vi "Read Step Data (Manual Mode).vi"(0 "VISA resource name":refnum<visa-resource-name>, 5 "Step (1)":i32=1 min=1 max=9 step=1 format="%2_0f", 11 "error in (no error)":errorcluster) -> (4 "VISA resource name out":refnum<visa-resource-name>, 6 "Test Meter Data Output":T1 {"Frequency (Hz)" format="%.1f"; "Voltage (V)" format="%.1f"; "RMS Current (A)" format="%.3f"; "Power (W)" format="%.1f"; "Peak Current (A)" format="%.1f"; "Power Factor" format="%.3f"}, 15 "error out":errorcluster)   [LabVIEW 2020]
doc: "Reads the Manual mode <B>Step data</B>. \n\nIn Manual Mode the output data cluster has the following data.\n\n1. Memory\n2. Frequency (Hz)\n3. Voltage (V)\n4. RMS Current (A)\n5. Peak Current (A)\n6. Power (W)\n7. Power Factor\n8. Status\n\nNote: This setting is supported for <B>Firmware Version 2.0</B> Only"
uses:
  <instrlib>/eec 6700/eec 6700.lvlib
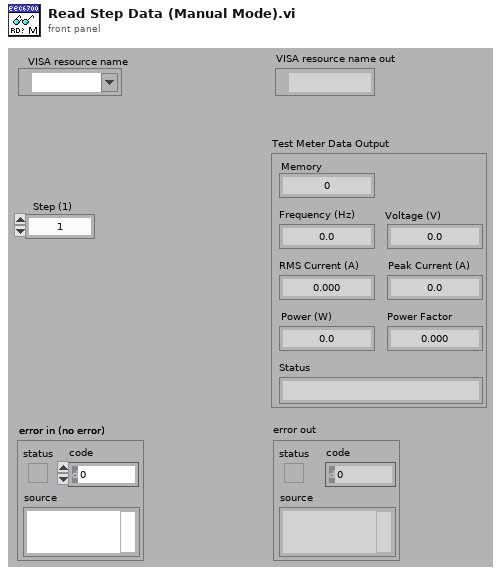
[diagram p1: front panel]
types:
  T1 = cluster{"Memory":i32, "Frequency (Hz)":dbl, "Voltage (V)":dbl, "RMS Current (A)":dbl, "Peak Current (A)":dbl, "Power (W)":dbl, "Power Factor":dbl, "Status":string}
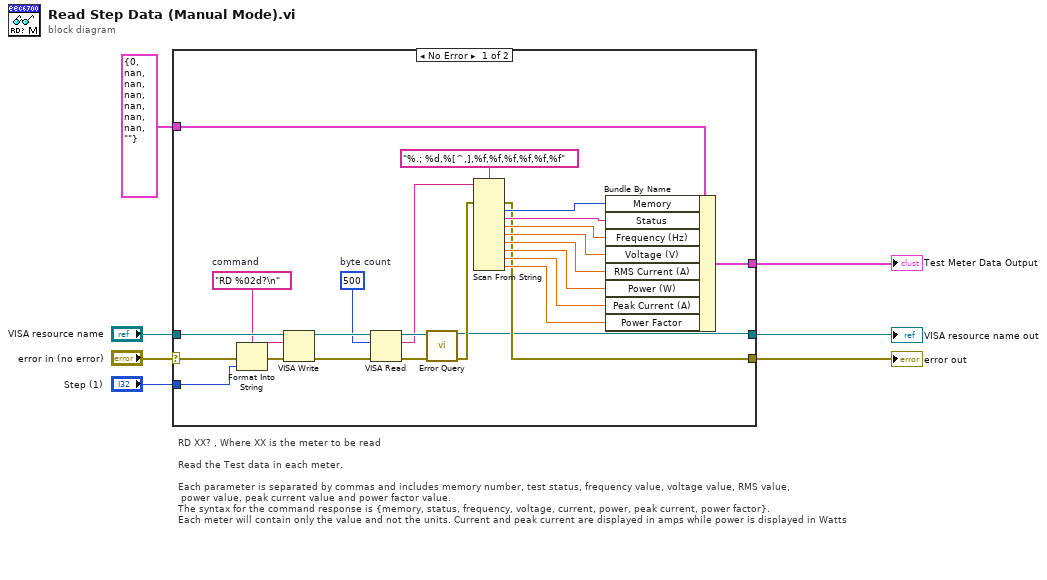
[diagram p0: block diagram]
diagram:
  # "RD XX? , Where XX is the meter to be read\n\nRead the Test data in each meter. \n\nEach parameter is separated by commas and includes memory number, test status, frequency value, voltage value, RMS value,\n power value, peak current value and power factor value. \nThe syntax for the command response is {memory, status, frequency, voltage, current, power, peak current, power factor}. \nEach meter will contain only the value and not the units. Current and peak current are displayed in amps while power is displayed in Watts"
  n1 = case shown="No Error" "error in (no error)" {
    selector: "error in (no error)" -> [w29 w35]
    tunnel: "VISA resource name" -> [w30 w36]
    tunnel: [w9 w36] -> w5
    tunnel: [w12 w35] -> w4
    tunnel: [w8 w34] -> w2
    tunnel: T1 {"Memory"=0, "Frequency (Hz)"=nan, "Voltage (V)"=nan, "RMS Current (A)"=nan, "Peak Current (A)"=nan, "Power (W)"=nan, "Power Factor"=nan, "Status"=""} ("Test Meter Data Output") -> [w10 w34]
    tunnel: "Step (1)" -> [w23 _]
    frame No Error {
      w25 = "RD %02d?\n"  # command
      w31 = u32 500  # byte count
      n2 = Format Into String(format string=w25, error in=w29, w23) -> (resulting string=w24:string, error out=w26:errorcluster)  [unwired: 1 in]
      n3 = VISA Write(VISA resource name=w30, write buffer=w24, error in (no error)=w26) -> (VISA resource name out=w33:refnum<visa-resource-name>, error out=w32:errorcluster)  [unwired: 1 out]
      n4 = VISA Read(VISA resource name=w33, byte count=w31, error in (no error)=w32) -> (VISA resource name out=w28:refnum<visa-resource-name>, read buffer=w11:string, error out=w27:errorcluster)  [unwired: 1 out]
      n5 = call <instrlib>:"Error Query.vi"("VISA resource name"=w28, "error in (no error)"=w27) -> ("VISA resource name out"=w9:refnum<visa-resource-name>, "error out"=w13:errorcluster)  [unwired: 10 in, 2 out]
      n6 = Scan From String(format string="%.; %d,%[^,],%f,%f,%f,%f,%f,%f", input string=w11, error in=w13) -> (error out=w12:errorcluster, output 1=w21:i32, output 2=w20:string, output 3=w19:dbl, output 4=w18:dbl, output 5=w17:dbl, output 6=w16:dbl, output 7=w15:dbl, output 8=w14:dbl)  [unwired: 9 in, 2 out]
      n7 = Bundle By Name(cluster=w10, "Memory"=w21, "Status"=w20, "Frequency (Hz)"=w19, "Voltage (V)"=w18, "RMS Current (A)"=w17, "Power (W)"=w16, "Peak Current (A)"=w15, "Power Factor"=w14) -> (w8:T1)
    }
    frame Error {
    }
  }
  "VISA resource name out" <- w5
  "error out" <- w4
  "Test Meter Data Output" <- w2
